vi "Close.vi"(8 "error in (no error)":errorcluster, 11 "State in":T1={"State"=enum."Idle", "Start Time"=timestamp(0 s since 1904-01-01), "Configuration"={"Cycle Period"=0.0, "Setpoint Entry"=0.0, "Output Device"=enum."Huber Ministat 230", "Huber Ministat 230 Settings"={"VISA resource name"="", "Simulated?"=FALSE}, "Lauda Settings"={"VISA resource name"="", "Simulated?"=FALSE, "Pump Power"=2}, "Julabo FP-50 Settings"={"VISA resource name"="", "Simulated?"=FALSE, "Pump Power"=2}, "Internal Control?"=FALSE, "Huber Unistat 410 Settings"={"VISA resource name"="", "Address"=0, "Simulated?"=FALSE}, "HOTCOIL Settings"={"VISA resource name"="", "Simulated?"=FALSE}}, "Current Time"=timestamp(0 s since 1904-01-01), "First Iteration"=FALSE, "Data"={"TCU Speed"=0.0, "Temperature"=0.0}, "Process Name"="", "TCU On?"=FALSE, "Output Error"=FALSE, "Start Log"=FALSE, "Power Level Changed"=FALSE} {"Configuration"."Huber Unistat 410 Settings"."Address" min=0 max=99 format="%02.0f"; "Configuration"."Julabo FP-50 Settings"."Pump Power" min=0 max=8 step=1; "Configuration"."Lauda Settings"."Pump Power" min=0 max=8 step=1}) -> (0 "error out":errorcluster, 3 "State out":T1={"State"=enum."Idle", "Start Time"=timestamp(0 s since 1904-01-01), "Configuration"={"Cycle Period"=0.0, "Setpoint Entry"=0.0, "Output Device"=enum."Huber Ministat 230", "Huber Ministat 230 Settings"={"VISA resource name"="", "Simulated?"=FALSE}, "Lauda Settings"={"VISA resource name"="", "Simulated?"=FALSE, "Pump Power"=2}, "Julabo FP-50 Settings"={"VISA resource name"="", "Simulated?"=FALSE, "Pump Power"=2}, "Internal Control?"=FALSE, "Huber Unistat 410 Settings"={"VISA resource name"="", "Address"=0, "Simulated?"=FALSE}, "HOTCOIL Settings"={"VISA resource name"="", "Simulated?"=FALSE}}, "Current Time"=timestamp(0 s since 1904-01-01), "First Iteration"=FALSE, "Data"={"TCU Speed"=0.0, "Temperature"=0.0}, "Process Name"="", "TCU On?"=FALSE, "Output Error"=FALSE, "Start Log"=FALSE, "Power Level Changed"=FALSE} {"Configuration"."Huber Unistat 410 Settings"."Address" min=0 max=99 format="%02.0f"; "Configuration"."Julabo FP-50 Settings"."Pump Power" min=0 max=8 step=1; "Configuration"."Lauda Settings"."Pump Power" min=0 max=8 step=1})   [LabVIEW 2021, in "TCU Module.lvlib" / "TCU Module Engine.lvlib"]
uses:
  TCU Module Engine.lvlib
  TCU State Cluster.ctl
  State Enum.ctl
  TCU Module Settings Cluster.ctl
  Output Devices.ctl
  Huber TCU/Huber Settings.ctl
  Lauda Integral XT-150 TCU/Lauda Settings.ctl
  Julabo Type 1 TCU/Julabo Type 1 TCU Folder/Julabo FP-50 Settings.ctl
  Huber Unistat 410 TCU/Huber Unistat 410 RS485 Settings.ctl
  HOTCOIL/HotCoil Settings.ctl
  Huber TCU/Huber Ministat 230 TCU.lvlib
  Lauda Integral XT-150 TCU/Lauda TCU.lvlib
  Julabo Type 1 TCU/Julabo Type 1 TCU Folder/Julabo Type FP-50 TCU.lvlib
  Huber Unistat 410 TCU/Huber Unistat 410 TCU.lvlib
  HOTCOIL/HotCoil.lvlib
  TCU Module.lvlib
panel:
  # "Output Instruments"
  # "Output Instruments"
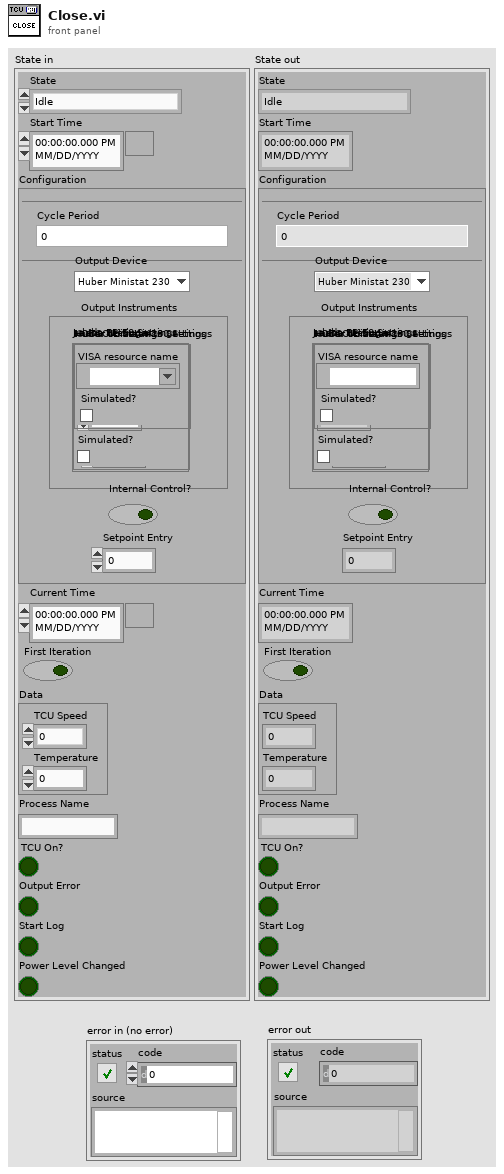
[diagram p1: front panel]
types:
  T1 = typedef "TCU Module.lvlib/TCU Module Engine.lvlib/TCU State Cluster.ctl" = cluster{"State":T2, "Start Time":timestamp, "Configuration":T3, "Current Time":timestamp, "First Iteration":bool, "Data":cluster{"TCU Speed":dbl, "Temperature":dbl}, "Process Name":string, "TCU On?":bool, "Output Error":bool, "Start Log":bool, "Power Level Changed":bool}
  T2 = typedef "TCU Module.lvlib/TCU Module Engine.lvlib/State Enum.ctl" = enum16{"Measuring", "Idle", "Paused"}
  T3 = typedef "TCU Module.lvlib/TCU Module Settings Cluster.ctl" = cluster{"Cycle Period":dbl, "Setpoint Entry":dbl, "Output Device":T4, "Huber Ministat 230 Settings":T5, "Lauda Settings":T6, "Julabo FP-50 Settings":T7, "Internal Control?":bool, "Huber Unistat 410 Settings":T8, "HOTCOIL Settings":T9}
  T4 = typedef "Output Devices.ctl" = enum16{"Default", "Huber Ministat 230", "Huber Unistat 410", "Lauda XT-150", "Julabo FP-50", "HotCoil"}
  T5 = typedef "Huber Ministat 230 TCU.lvlib/Huber Settings.ctl" = cluster{"VISA resource name":refnum<visa-resource-name>, "Simulated?":bool}
  T6 = typedef "Lauda TCU.lvlib/Lauda Settings.ctl" = cluster{"VISA resource name":refnum<visa-resource-name>, "Simulated?":bool, "Pump Power":i32}
  T7 = typedef "Julabo Type FP-50 TCU.lvlib/Julabo FP-50 Settings.ctl" = cluster{"VISA resource name":refnum<visa-resource-name>, "Simulated?":bool, "Pump Power":i32}
  T8 = typedef "Huber Unistat 410 TCU.lvlib/Huber Unistat 410 RS485 Settings.ctl" = cluster{"VISA resource name":refnum<visa-resource-name>, "Address":i8, "Simulated?":bool}
  T9 = typedef "HotCoil.lvlib/HotCoil Settings.ctl" = cluster{"VISA resource name":refnum<visa-resource-name>, "Simulated?":bool}
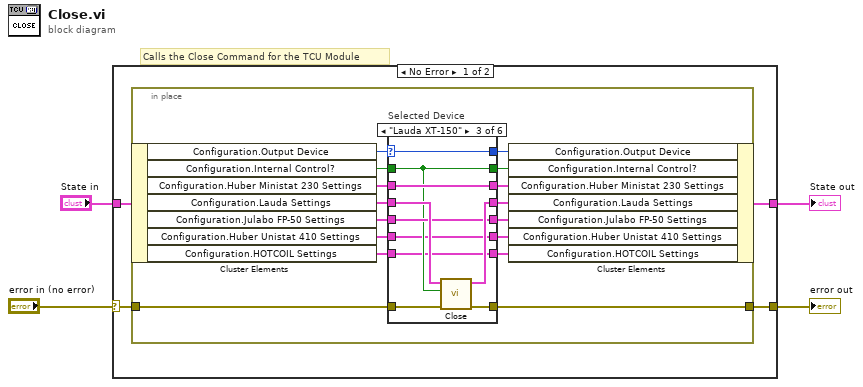
[diagram p0: block diagram]
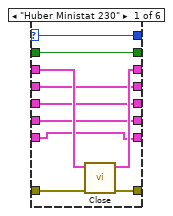
[diagram p2: hidden frame]
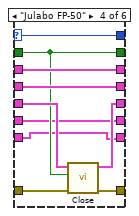
[diagram p4: hidden frame]
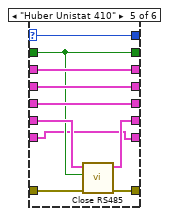
[diagram p5: hidden frame]
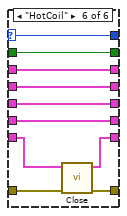
[diagram p6: hidden frame]
diagram:
  # "Calls the Close Command for the TCU Module"
  n1 = case shown="No Error" "error in (no error)" {
    selector: "error in (no error)" -> [w7 w84]
    tunnel: [w8 w84] -> w3
    tunnel: "State in" -> [w6 w83]
    tunnel: [w5 w83] -> w1
    frame No Error {
      n2 = in-place {
        in-place-border: [w24] -> w8
        in-place-border: w7 -> [w23]
        n3 = in-place-cluster #1(w6) -> ("Configuration.Output Device"=w14:T4, "Configuration.Internal Control?"=w13:bool, "Configuration.Huber Ministat 230 Settings"=w22:T5, "Configuration.Lauda Settings"=w21:T6, "Configuration.Julabo FP-50 Settings"=w20:T7, "Configuration.Huber Unistat 410 Settings"=w16:T8, "Configuration.HOTCOIL Settings"=w10:T9)
        n4 = case "Selected Device" shown="\"Lauda XT-150\"" w14 {
          selector: w14 -> [w26 w36 w44 w54 w64 w76]
          tunnel: w22 -> [w32 w41 w52 w62 w72 w82]
          tunnel: [w34 w42 w49 w59 w66 w78] -> w24
          tunnel: w23 -> [w33 w42 w48 w60 w67 w79]
          tunnel: [w31 w41 w52 w62 w72 w82] -> w19
          tunnel: w21 -> [w30 w40 w51 w61 w71 w81]
          tunnel: [w30 w40 w50 w61 w71 w81] -> w18
          tunnel: [w29 w39 w47 w57 w70 w80] -> w17
          tunnel: w20 -> [w29 w39 w47 w58 w70 w80]
          tunnel: w13 -> [w27 w37 w46 w56 w68 w75]
          tunnel: w16 -> [w28 w38 w45 w55 w69 w77]
          tunnel: [w28 w38 w45 w55 w65 w77] -> w15
          tunnel: [w26 w36 w44 w54 w64 w76] -> w12
          tunnel: [w27 w37 w46 w56 w68 w75] -> w11
          tunnel: w10 -> [w25 w35 w43 w53 w63 w74]
          tunnel: [w25 w35 w43 w53 w63 w73] -> w9
          frame "Huber Ministat 230" {
            n5 = call "Close.vi"("error in (no error)"=w33, "Huber Settings"=w32) -> ("error out"=w34:errorcluster, "Huber Settings"=w31:T5)  [unwired: 8 in]
          }
          frame "Default", Default {
          }
          frame "Lauda XT-150" {
            n6 = call "Close.vi"("error in (no error)"=w48, "Internal?"=w46, "Lauda  Settings"=w51) -> ("error out"=w49:errorcluster, "Lauda Settings"=w50:T6)  [unwired: 7 in]
          }
          frame "Julabo FP-50" {
            n7 = call "Close.vi"("error in (no error)"=w60, "Internal?"=w56, "Julabo Fp-50 Settings"=w58) -> ("error out"=w59:errorcluster, "Julabo FP-50 Settings"=w57:T7)  [unwired: 7 in]
          }
          frame "Huber Unistat 410" {
            n8 = call "Close RS485.vi"("error in (no error)"=w67, "Internal?"=w68, "Huber Unistat 410 Settings"=w69) -> ("error out"=w66:errorcluster, "Huber Unistat 410 Settings"=w65:T8)  [unwired: 7 in]
          }
          frame "HotCoil" {
            n9 = call "Close.vi"("error in (no error)"=w79, "HOTCOIL Settings"=w74) -> ("error out"=w78:errorcluster, "HOTCOIL Settings"=w73:T9)  [unwired: 8 in]
          }
        }
        n10 = in-place-cluster #1("Configuration.Output Device"=w12, "Configuration.Internal Control?"=w11, "Configuration.Huber Ministat 230 Settings"=w19, "Configuration.Lauda Settings"=w18, "Configuration.Julabo FP-50 Settings"=w17, "Configuration.Huber Unistat 410 Settings"=w15, "Configuration.HOTCOIL Settings"=w9) -> (w5:T1)
      }
    }
    frame Error {
    }
  }
  "error out" <- w3
  "State out" <- w1
